vi "DelayGenerator.vi"(11 "Delay(cycles)":u32) -> (3 "Trigger":bool)   [LabVIEW 2018]
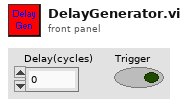
[diagram p1: front panel]
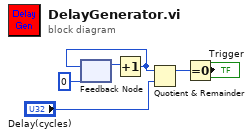
[diagram p0: block diagram]
diagram:
  n1 = feedback #1(0) -> (w2:i32)
  n2 = Increment(x=w2) -> (x+1=w3:i32)
  n3 = feedback-in #1(w3) -> ()
  n4 = Quotient & Remainder(x=w3, y="Delay(cycles)") -> (x-y*floor(x/y)=w5:u32)  [unwired: 1 out]
  n5 = Equal To 0?(x=w5) -> (x = 0?=→"Trigger":bool)
